vi "LTVDiffDriveCtrl_Calculate.vi"(4 "Ref Right Velocity":dbl, 5 "Left Velocity":dbl, 6 "Ref Left Velocity":dbl, 7 "Right Velocity":dbl, 9 "RefPose":T1={"TRANSLATION"={"X"=0.0, "Y"=0.0}, "ROTATION"={"VALUE"=0.0, "COS"=1.0, "SIN"=0.0}} {"ROTATION"."SIN" format="%13.4f"; "ROTATION"."COS" format="%13.4f"; "ROTATION"."VALUE" format="%13.4f"; "TRANSLATION"."Y" format="%14.3f"; "TRANSLATION"."X" format="%14.3f"}, 10 "CurrentPose":T1={"TRANSLATION"={"X"=0.0, "Y"=0.0}, "ROTATION"={"VALUE"=0.0, "COS"=1.0, "SIN"=0.0}} {"ROTATION"."SIN" format="%13.4f"; "ROTATION"."COS" format="%13.4f"; "ROTATION"."VALUE" format="%13.4f"; "TRANSLATION"."Y" format="%14.3f"; "TRANSLATION"."X" format="%14.3f"}, 11 "in LTVDiffDriveCtrl":T4) -> (0 "Error":bool, 1 "Right Voltage":dbl, 2 "Left Voltage":dbl, 3 "out LTVDiffDriveCtrl":T4)   [LabVIEW 2019, in "Trajectory_Library.lvlib"]
doc: "Create implicit model follower\n\nInputs:\n - A < states, states > -- Continuous system matrix of the plant being controlled.\n - B < states, inputs > -- Continuous input matrix of the plant being controlled.\n - A_Ref < states, states > -- Continuous system matrix whose dymanics should be followed.\n - B_Ref < states, inputs > -- Continuous input matrix x whose dymanics should be followed.\n\nOutputs:\n - Error -- If TRUE, an error occured."
uses:
  Trajectory_Library.lvlib
  <vilib>/Analysis/Matrix/NI_Matrix.lvlib
  <vilib>/Analysis/Matrix/Numeric/Subtract/Subtract - RM,RM.vi
  TypeDef/LTV_DIFF_DRIVE_CTRL_STATE_ENUM.ctl
  <vilib>/Analysis/NI_AALBase.lvlib
  <vilib>/Analysis/baseanly.llb/Real A x B.vi
  <vilib>/Analysis/Matrix/Datatypes/RealMatrix.ctl
  TypeDef/TRANSLATION2D.ctl
  TypeDef/ROTATION2D.ctl
  TypeDef/POSE2D.ctl
  TypeDef/FUNCTION_GENERATOR_MATRIX.ctl
  TypeDef/LTV_DIFF_DRIVE_CTRL.ctl
panel:
  # "< 5, 1 >"
  # "< 5, 1 >"
  # "< 5, 1 >"
  # "< 5, 1 >"
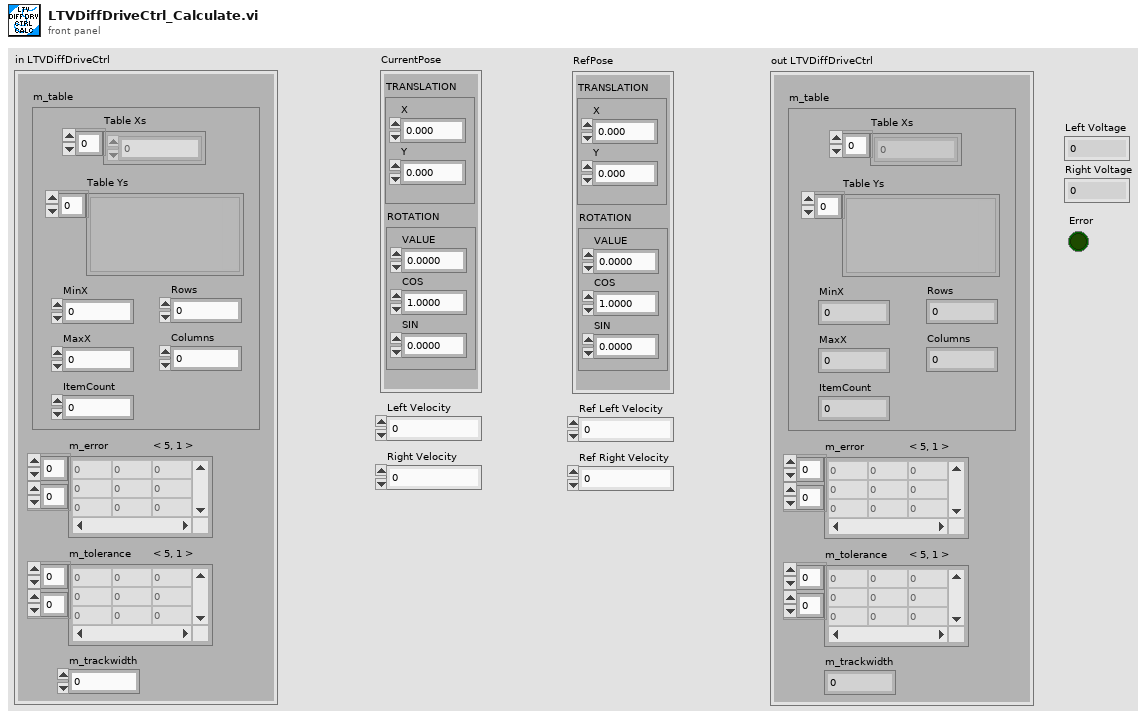
[diagram p1: front panel]
types:
  T1 = typedef "Trajectory_Library.lvlib/POSE2D.ctl" = cluster{"TRANSLATION":T2, "ROTATION":T3}
  T2 = typedef "Trajectory_Library.lvlib/TRANSLATION2D.ctl" = cluster{"X":dbl, "Y":dbl}
  T3 = typedef "Trajectory_Library.lvlib/ROTATION2D.ctl" = cluster{"VALUE":dbl, "COS":dbl, "SIN":dbl}
  T4 = typedef "Trajectory_Library.lvlib/LTV_DIFF_DRIVE_CTRL.ctl" = cluster{"m_table":T5, "m_error":T6, "m_tolerance":T6, "m_trackwidth":dbl}
  T5 = typedef "Trajectory_Library.lvlib/FUNCTION_GENERATOR_MATRIX.ctl" = cluster{"Table Xs":dbl[], "Table Ys":variant[], "MinX":dbl, "MaxX":dbl, "ItemCount":i32, "Rows":i32, "Columns":i32}
  T6 = typedef "NI_Matrix.lvlib/RealMatrix.ctl" = dbl[][]
  T7 = typedef "Trajectory_Library.lvlib/LTV_DIFF_DRIVE_CTRL_STATE_ENUM.ctl" = enum16{"X_POS", "Y_POS", "HEADING", "LEFT_VEL", "RIGHT_VEL"}
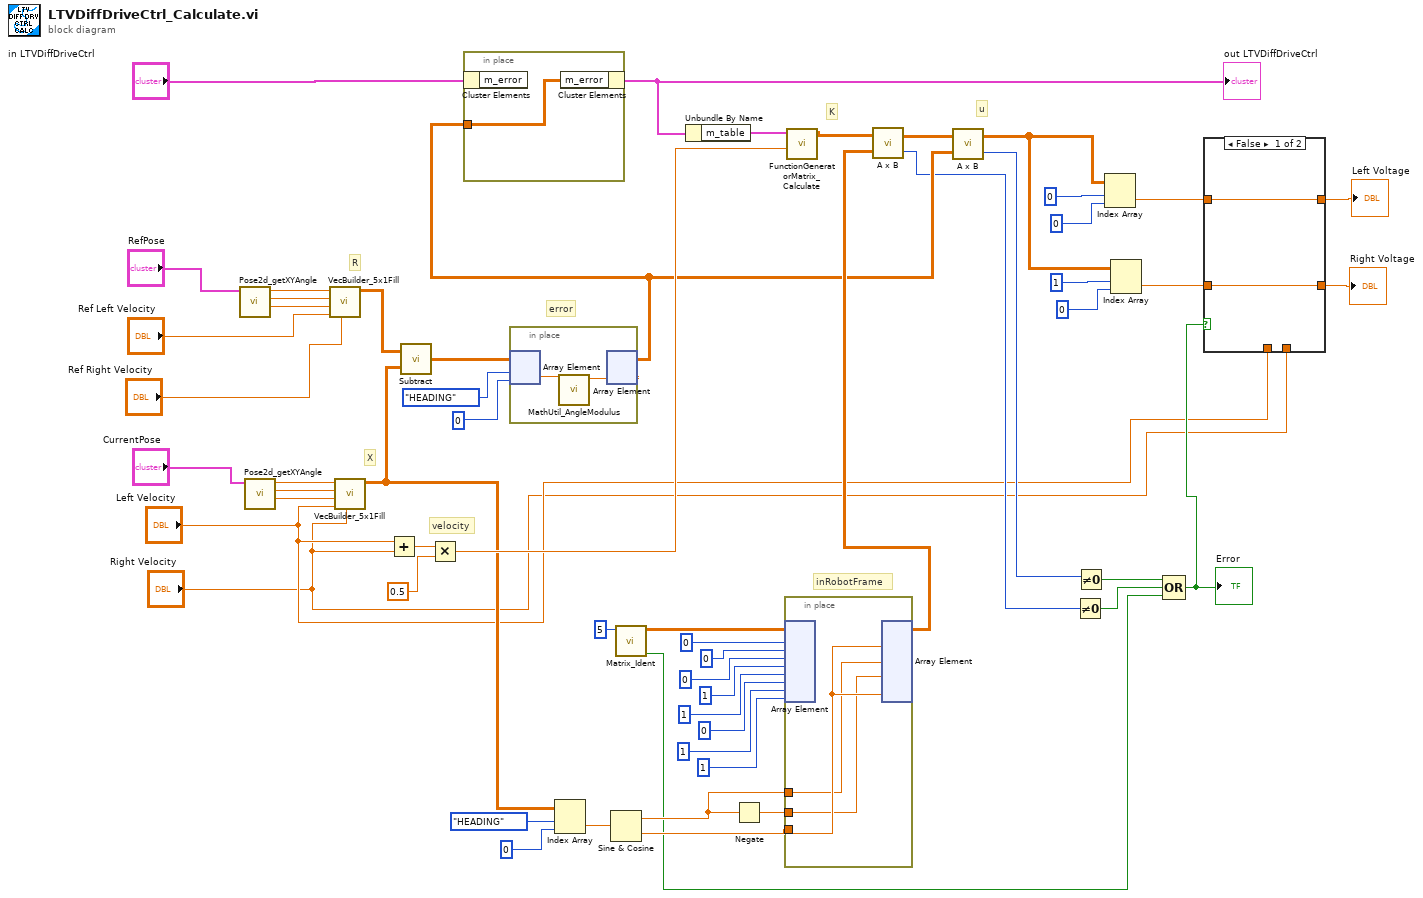
[diagram p0: block diagram]
diagram:
  # "error"
  # "u"
  # "inRobotFrame"
  # "K"
  # "velocity"
  # "R"
  # "X"
  n1 = call "Pose2d_getXYAngle.vi"("in POSE"="RefPose") -> ("Angle"=w50:dbl, "Y"=w51:dbl, "X"=w52:dbl)  [unwired: 8 in]
  n2 = call "Pose2d_getXYAngle.vi"("in POSE"="CurrentPose") -> ("Angle"=w55:dbl, "Y"=w56:dbl, "X"=w57:dbl)  [unwired: 8 in]
  n3 = call "VecBuilder_5x1Fill.vi"("R4"="Ref Right Velocity", "R3"="Ref Left Velocity", "R2"=w50, "R1"=w51, "R0"=w52) -> ("output matrix"=w46:T6)  [unwired: 6 in]
  n4 = call "VecBuilder_5x1Fill.vi"("R4"="Right Velocity", "R3"="Left Velocity", "R2"=w55, "R1"=w56, "R0"=w57) -> ("output matrix"=w26:T6)  [unwired: 6 in]
  n5 = Add(x="Left Velocity", y="Right Velocity") -> (x+y=w42:dbl)
  n6 = call-poly <vilib>:"Subtract.vi"("Real Matrix B"=w26, "Real Matrix A"=w46) -> ("A - B"=w45:T6)
  n7 = Multiply(x=w42, y=0.5) -> (x*y=w38:dbl)
  n8 = in-place {
    n9 = in-place-array #1(w45, LTV_DIFF_DRIVE_CTRL_STATE_ENUM."HEADING" ("LTV_DIFF_DRIVE_CTRL_STATE"), 0 ("disabled index (col)")) -> (w60:dbl)
    n10 = call "MathUtil_AngleModulus.vi"("InputAngle"=w60) -> ("ModulsAngle"=w59:dbl)  [unwired: 10 in]
    n11 = in-place-array #1(w59) -> (w18:T6)  [unwired: 2 out]
  }
  n12 = in-place {
    in-place-border: w18 -> [w61]
    n13 = in-place-cluster #2("in LTVDiffDriveCtrl") -> ()  [unwired: 1 out]
    n14 = in-place-cluster #2("m_error"=w61) -> (w40:T4)
  }
  "out LTVDiffDriveCtrl" <- w40
  n15 = Index Array(array=w26, index (row)=LTV_DIFF_DRIVE_CTRL_STATE_ENUM."HEADING" ("LTV_DIFF_DRIVE_CTRL_STATE"), index (col)=0 ("disabled index (col)")) -> (element=w25:dbl)
  n16 = Sine & Cosine(0:w25) -> (1:w23:dbl, 2:w24:dbl)
  n17 = call "Matrix_Ident.vi"("Size"=5) -> ("Error"=w8:bool, "output matrix"=w37:T6)  [unwired: 9 in]
  n18 = Unbundle By Name(w40) -> ("m_table"=w39:T5)
  n19 = Negate(x=w23) -> (-x=w22:dbl)
  n20 = in-place {
    in-place-border: w24 -> [w64]
    in-place-border: w23 -> [w63]
    in-place-border: w22 -> [w62]
    n21 = in-place-array #3(w37, 0 ("disabled index (row)"), 0 ("disabled index (col)"), 0 ("disabled index (row)"), 1 ("disabled index (col)"), 1 ("disabled index (row)"), 0 ("disabled index (col)"), 1 ("disabled index (row)"), 1 ("disabled index (col)")) -> ()  [unwired: 4 out]
    n22 = in-place-array #3(w64, w63, w62, w64) -> (w20:T6)  [unwired: 8 out]
  }
  n23 = call "FunctionGeneratorMatrix_Calculate.vi"("Input Value"=w38, "FUNCTION_GENERATOR_MATRIX"=w39) -> ("Output Matrix"=w21:T6)  [unwired: 9 in]
  n24 = call-poly <vilib>:"A x B.vi"("B"=w20, "A"=w21) -> ("error"=w9:i32, "A x B"=w19:T6)
  n25 = call-poly <vilib>:"A x B.vi"("B"=w18, "A"=w19) -> ("error"=w10:i32, "A x B"=w13:T6)
  n26 = Not Equal To 0?(x=w9) -> (x != 0?=w11:bool)
  n27 = Not Equal To 0?(x=w10) -> (x != 0?=w12:bool)
  n28 = Index Array(array=w13, index (row)=0, index (col)=0 ("disabled index (col)")) -> (element=w6:dbl)
  n29 = Index Array(array=w13, index (row)=1, index (col)=0 ("disabled index (col)")) -> (element=w5:dbl)
  n30 = Compound Arithmetic op=OR(w12, w11, w8) -> (w7:bool)
  "Error" <- w7
  n31 = case shown="False" w7 {
    tunnel: w6 -> [w66 _]
    tunnel: w5 -> [w65 _]
    tunnel: [w66 w67] -> w4
    tunnel: [w65 w68] -> w3
    tunnel: "Right Velocity" -> [_ w68]
    tunnel: "Left Velocity" -> [_ w67]
    frame False {
    }
    frame True {
    }
  }
  "Left Voltage" <- w4
  "Right Voltage" <- w3
